vi "SimonGame.vi"() -> ()   [LabVIEW 2024]
uses:
  state machine variables.ctl
  state machine states.ctl
  state machine controller.ctl
panel:
  in  "Button 4":bool
  in  "Button3":bool
  in  "Button 2":bool
  in  "Button 1":bool
  out "Round":dbl
  out "Score":dbl
  # "Score"
  # "Level"
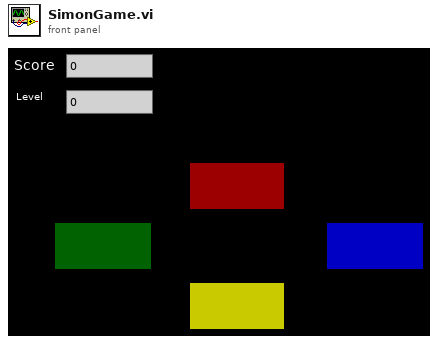
[diagram p1: front panel]
types:
  T1 = typedef "state machine states.ctl" = enum16{"Initialize", "update display", "Show sequence", "User response", "update data", ""}
  T2 = typedef "state machine variables.ctl" = cluster{"Sequence":dbl[], "Score":dbl, "Round":dbl}
  T3 = typedef "VI Communication.ctl" = cluster{"Queue":refnum<queue>, "Path":path, "Score":dbl, "Level":dbl}
  T4 = enum8{"Enabled", "Disabled", "Disabled and Grayed Out"}
  T5 = typedef "state machine controller.ctl" = cluster{"State Machine State":string, "Difficulty":dbl, "Login User Name":string, "Login User Passwd":string}
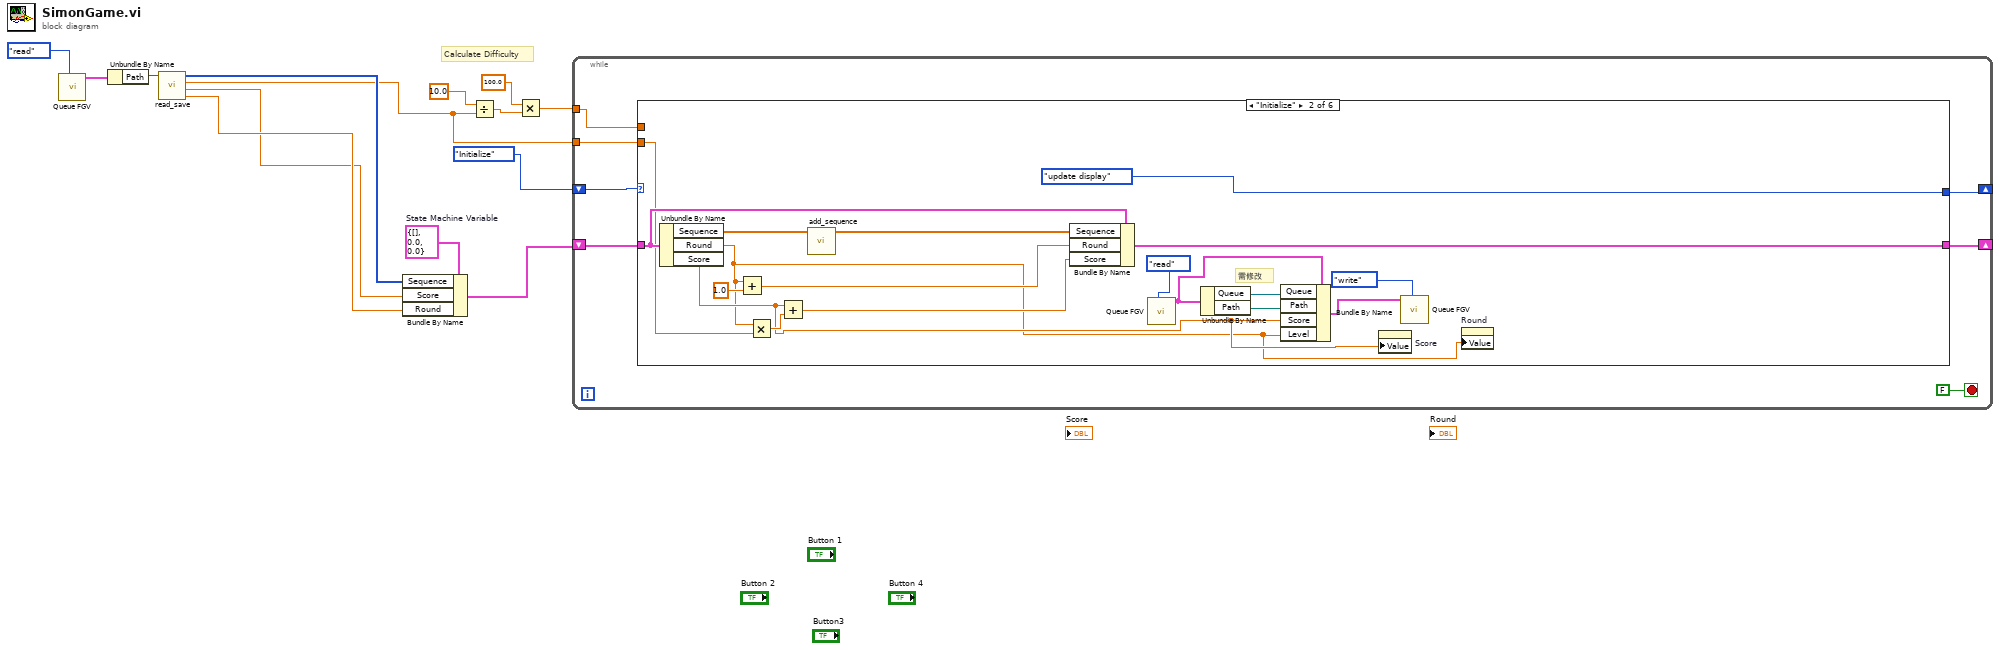
[diagram p0: block diagram]
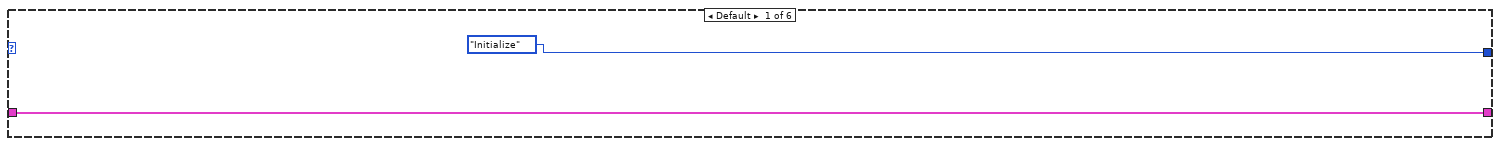
[diagram p2: hidden frame]
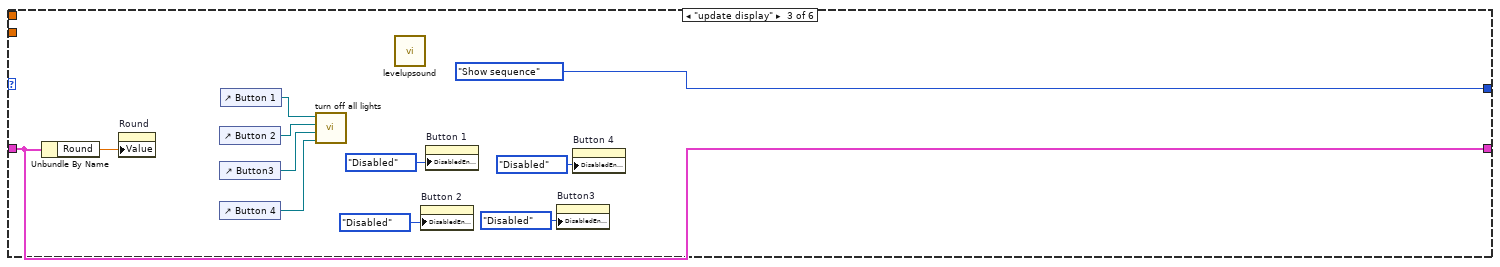
[diagram p3: hidden frame]
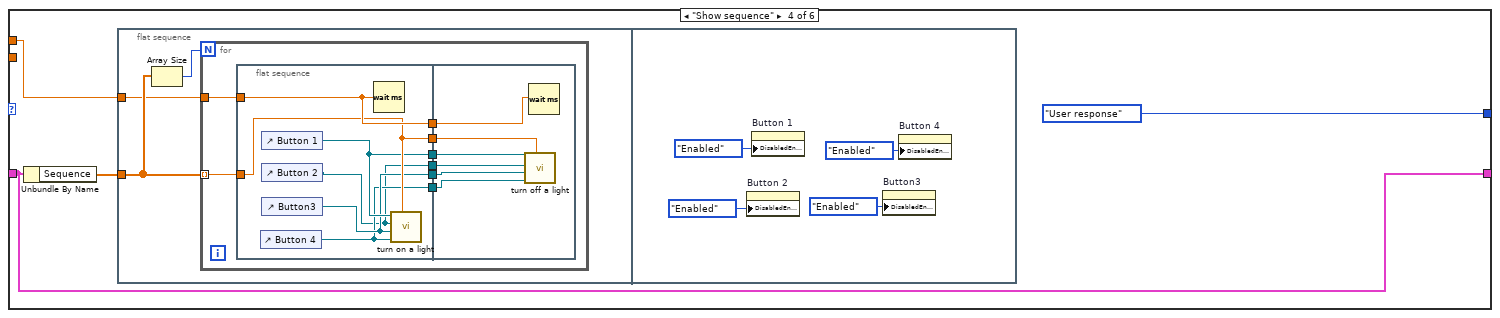
[diagram p4: hidden frame]
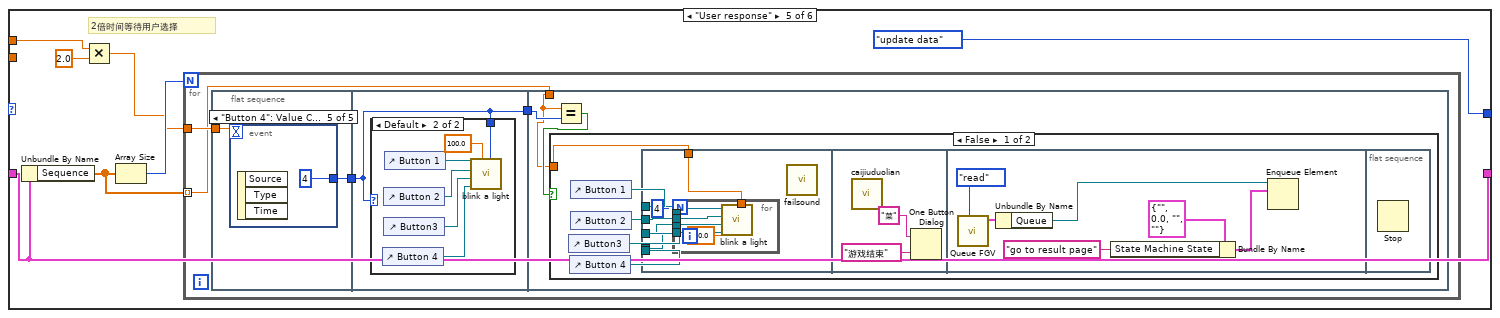
[diagram p5: hidden frame]
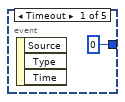
[diagram p6: hidden frame]
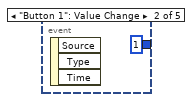
[diagram p7: hidden frame]
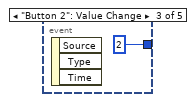
[diagram p8: hidden frame]
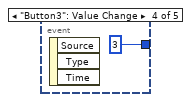
[diagram p9: hidden frame]
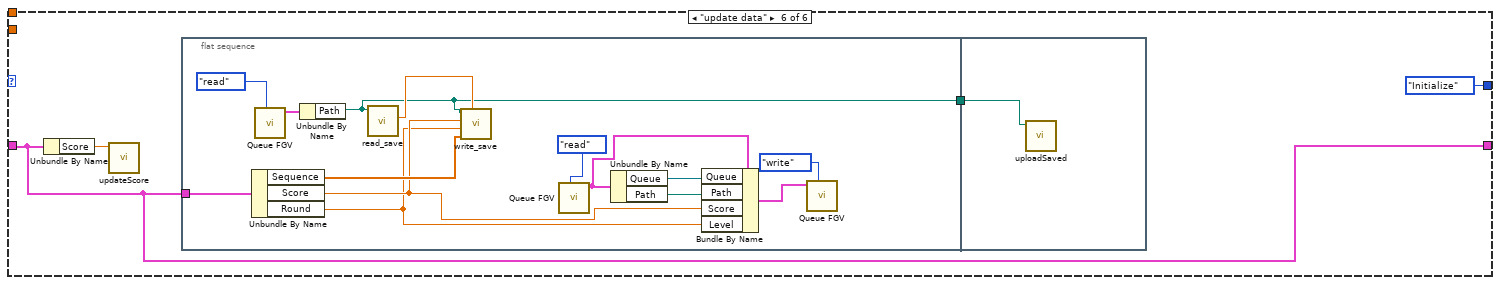
[diagram p12: hidden frame]
diagram:
  w9 = T2 {"Sequence"=[], "Score"=0.0, "Round"=0.0}  # State Machine Variable
  # "Calculate Difficulty"
  n1 = call "Queue FGV.vi"("Enum"=enum16{"read", "write"}."read") -> ("VI Communication Out"=w5:T3)  [unwired: 10 in]
  n2 = Unbundle By Name(w5) -> ("Path"=w4:path)
  n3 = call "read_save.vi"("save file path"=w4) -> ("Level"=w3:dbl, "Score"=w2:dbl, "Difficulty"=w1:dbl, "Sequence Array"=w7:i32[])  [unwired: 6 in, 1 out]
  n4 = Bundle By Name(cluster=w9, "Sequence"=w7, "Score"=w2, "Round"=w3) -> (w8:T2)
  n5 = Divide(x=10.0, y=w1) -> (x/y=w12:dbl)
  n6 = Multiply(x=100.0, y=w12) -> (x*y=w11:dbl)
  n7 = while {
    shift-right: [w17] -> _
    shift-left: w8 -> [w21]
    shift-right: [w19] -> _
    shift-left: state_machine_states."Initialize" -> [w20]
    tunnel: w11 -> [w18]
    tunnel: w1 -> [w16]
    stop <- FALSE stop-if-true
    n8 = case shown="\"Initialize\"" w20 {
      tunnel: w21 -> [w23 w40 w52 w53 w84 w137]
      tunnel: [w23 w39 w52 w53 w84 w137] -> w17
      tunnel: [state_machine_states."Initialize" ("Enum") state_machine_states."update display" ("Enum") state_machine_states."Show sequence" ("Enum") state_machine_states."User response" ("Enum") state_machine_states."update data" ("Enum") state_machine_states."Initialize" ("Enum")] -> w19
      tunnel: w18 -> [_ _ _ w55 w86 _]
      tunnel: w16 -> [_ w34 _ _ _ _]
      frame Default {
      }
      frame "Initialize" {
        # "需修改"
        n9 = Unbundle By Name(w40) -> ("Sequence"=w41:dbl[], "Round"=w24:dbl, "Score"=w25:dbl)
        n10 = Add(x=w24, y=1.0) -> (x+y=w28:dbl)
        n11 = Multiply(x=w24, y=w34) -> (x*y=w35:dbl)
        n12 = Add(x=w25, y=w35) -> (x+y=w27:dbl)
        n13 = call "add_sequence.vi"("sequence in"=w41) -> ("sequence out"=w38:dbl[])  [unwired: 9 in, 1 out]
        n14 = Bundle By Name(cluster=w40, "Sequence"=w38, "Round"=w28, "Score"=w27) -> (w39:T2)
        n15 = call "Queue FGV.vi"("Enum"=enum16{"read", "write"}."read") -> ("VI Communication Out"=w32:T3)  [unwired: 10 in]
        n16 = Unbundle By Name(w32) -> ("Queue"=w30:refnum<queue>, "Path"=w29:path)
        n17 = Bundle By Name(cluster=w32, "Queue"=w30, "Path"=w29, "Score"=w25, "Level"=w24) -> (w26:T3)
        n18 = property on="Score" class="DigNum (strict)"("Value"=w25) -> ()  [unwired: 2 in, 2 out]
        n19 = call "Queue FGV.vi"("Enum"=enum16{"read", "write"}."write", "VI Communication In"=w26) -> ()  [unwired: 9 in, 1 out]
        n20 = property on="Round" class="DigNum (strict)"("Value"=w24) -> ()  [unwired: 2 in, 2 out]
      }
      frame "update display" {
        n21 = Unbundle By Name(w52) -> ("Round"=w51:dbl)
        n22 = property on="Round" class="DigNum (strict)"("Value"=w51) -> ()  [unwired: 2 in, 2 out]
        n23 = control-ref of="Button 2"() -> (w48:refnum<vi>)
        n24 = control-ref of="Button3"() -> (w47:refnum<vi>)
        n25 = control-ref of="Button 4"() -> (w46:refnum<vi>)
        n26 = control-ref of="Button 1"() -> (w49:refnum<vi>)
        n27 = call "turn off all lights.vi"("Button 4"=w46, "Button 3"=w47, "Button 2"=w48, "Button 1"=w49) -> ()  [unwired: 7 in, 1 out]
        n28 = call "levelupsound.vi"() -> ()  [unwired: 11 in, 1 out]
        n29 = property on="Button 2" class="Bool"("DisabledEnum"=T4."Disabled" ("Disabled")) -> ()  [unwired: 2 in, 2 out]
        n30 = property on="Button 1" class="Bool"("DisabledEnum"=T4."Disabled" ("Disabled")) -> ()  [unwired: 2 in, 2 out]
        n31 = property on="Button3" class="Bool"("DisabledEnum"=T4."Disabled" ("Disabled")) -> ()  [unwired: 2 in, 2 out]
        n32 = property on="Button 4" class="Bool"("DisabledEnum"=T4."Disabled" ("Disabled")) -> ()  [unwired: 2 in, 2 out]
      }
      frame "Show sequence" {
        n33 = Unbundle By Name(w53) -> ("Sequence"=w56:dbl[])
        n34 = flat-sequence {
          tunnel: w56 -> [w58]
          tunnel: w55 -> [w57]
          frame #0 {
            n35 = Array Size(array=w58) -> (size(s)=w59:i32)
            n36 = for {
              N: w59 -> [_]
              tunnel: w58 -> [w67] mode=indexing
              tunnel: w57 -> [w66]
              n37 = flat-sequence {
                tunnel: w67 -> [w72]
                tunnel: w66 -> [w73]
                tunnel: [w73] -> w65
                tunnel: [w72] -> w64
                tunnel: [w71] -> w63
                tunnel: [w70] -> w62
                tunnel: [w69] -> w61
                tunnel: [w68] -> w60
                tunnel: w65 -> [w79]
                tunnel: w64 -> [w78]
                tunnel: w63 -> [w77]
                tunnel: w62 -> [w76]
                tunnel: w61 -> [w75]
                tunnel: w60 -> [w74]
                frame #0 {
                  n38 = control-ref of="Button 4"() -> (w69:refnum<vi>)
                  n39 = control-ref of="Button 1"() -> (w71:refnum<vi>)
                  n40 = control-ref of="Button 2"() -> (w68:refnum<vi>)
                  n41 = control-ref of="Button3"() -> (w70:refnum<vi>)
                  n42 = Wait (ms)(milliseconds to wait=w73) -> ()  [unwired: 1 out]
                  n43 = call "turn on a light.vi"("Which Button?"=w72, "Button 4"=w69, "Button 3"=w70, "Button 2"=w68, "Button 1"=w71) -> ()  [unwired: 6 in, 1 out]
                }
                frame #1 {
                  n44 = call "turn off a light.vi"("Which Button?"=w78, "Button 4"=w75, "Button 3"=w76, "Button 2"=w74, "Button 1"=w77) -> ()  [unwired: 6 in, 1 out]
                  n45 = Wait (ms)(milliseconds to wait=w79) -> ()  [unwired: 1 out]
                }
              }
            }
          }
          frame #1 {
            n46 = property on="Button 2" class="Bool"("DisabledEnum"=T4."Enabled" ("Disabled")) -> ()  [unwired: 2 in, 2 out]
            n47 = property on="Button 1" class="Bool"("DisabledEnum"=T4."Enabled" ("Disabled")) -> ()  [unwired: 2 in, 2 out]
            n48 = property on="Button3" class="Bool"("DisabledEnum"=T4."Enabled" ("Disabled")) -> ()  [unwired: 2 in, 2 out]
            n49 = property on="Button 4" class="Bool"("DisabledEnum"=T4."Enabled" ("Disabled")) -> ()  [unwired: 2 in, 2 out]
          }
        }
      }
      frame "User response" {
        # "2倍时间等待用户选择"
        n50 = Unbundle By Name(w84) -> ("Sequence"=w88:dbl[])
        n51 = Multiply(x=w86, y=2.0) -> (x*y=w87:dbl)
        n52 = Array Size(array=w88) -> (size(s)=w89:i32)
        n53 = for {
          N: w89 -> [_]
          tunnel: w88 -> [w92] mode=indexing
          tunnel: w87 -> [w94]
          n54 = flat-sequence {
            tunnel: w94 -> [w96]
            tunnel: [w95] -> w93
            tunnel: w93 -> [w102]
            tunnel: [w102] -> w91
            tunnel: w92 -> [w109]
            tunnel: w91 -> [w111]
            frame #0 {
              n55 = event shown="[4] \"Button 4\": Value Change" {
                selector: _ -> [_ _ _ _ _]
                dyn-events: _ -> [_ _ _ _ _]
                timeout: w96 -> [_ _ _ _ _]
                tunnel: [u32 0 1 2 3 u32 4] -> w95
                event Timeout {
                  n56 = event-data() -> ()  [unwired: 1 in, 3 out]
                }
                event "Button 1": Value Change {
                  n57 = event-data() -> ()  [unwired: 1 in, 3 out]
                }
                event "Button 2": Value Change {
                  n58 = event-data() -> ()  [unwired: 1 in, 3 out]
                }
                event "Button3": Value Change {
                  n59 = event-data() -> ()  [unwired: 1 in, 3 out]
                }
                event "Button 4": Value Change {
                  n60 = event-data() -> ()  [unwired: 1 in, 3 out]
                }
              }
            }
            frame #1 {
              n61 = case shown="Default" w102 {
                tunnel: w102 -> [_ w108]
                frame 0 {
                }
                frame Default {
                  n62 = control-ref of="Button 4"() -> (w104:refnum<vi>)
                  n63 = control-ref of="Button 2"() -> (w106:refnum<vi>)
                  n64 = control-ref of="Button3"() -> (w105:refnum<vi>)
                  n65 = control-ref of="Button 1"() -> (w107:refnum<vi>)
                  n66 = call "blink a light.vi"("Whcih Button?"=w108, "Blink Time"=100.0, "Button 4"=w104, "Button 3"=w105, "Button 2"=w106, "Button 1"=w107) -> ()  [unwired: 5 in, 1 out]
                }
              }
            }
            frame #2 {
              n67 = Equal?(x=w109, y=w111) -> (x = y?=w110:bool)
              n68 = case shown="False" w110 {
                tunnel: w109 -> [w116 _]
                frame False {
                  n69 = control-ref of="Button3"() -> (w113:refnum<vi>)
                  n70 = control-ref of="Button 4"() -> (w112:refnum<vi>)
                  n71 = control-ref of="Button 1"() -> (w115:refnum<vi>)
                  n72 = control-ref of="Button 2"() -> (w114:refnum<vi>)
                  n73 = flat-sequence {
                    tunnel: w116 -> [w122]
                    tunnel: w115 -> [w119]
                    tunnel: w114 -> [w118]
                    tunnel: w113 -> [w120]
                    tunnel: [w121] -> _
                    tunnel: w112 -> [w121]
                    frame #0 {
                      n74 = for {
                        N: 4 -> [_]
                        tunnel: w122 -> [w128]
                        tunnel: w121 -> [w127]
                        tunnel: w120 -> [w126]
                        tunnel: w119 -> [w125]
                        tunnel: w118 -> [w124]
                        n75 = call "blink a light.vi"("Whcih Button?"=w128, "Blink Time"=200.0, "Button 4"=w127, "Button 3"=w126, "Button 2"=w124, "Button 1"=w125) -> ()  [unwired: 5 in, 1 out]
                      }
                      n76 = call "failsound.vi"() -> ()  [unwired: 11 in, 1 out]
                    }
                    frame #1 {
                      n77 = call "caijiuduolian.vi"() -> ()  [unwired: 11 in, 1 out]
                      n78 = One Button Dialog(message="菜", button name ("OK")="游戏结束") -> ()  [unwired: 1 out]
                    }
                    frame #2 {
                      n79 = call "Queue FGV.vi"("Enum"=enum16{"read", "write"}."read") -> ("VI Communication Out"=w131:T3)  [unwired: 10 in]
                      n80 = Unbundle By Name(w131) -> ("Queue"=w135:refnum<queue>)
                      n81 = Bundle By Name(cluster=T5 {"State Machine State"="", "Difficulty"=0.0, "Login User Name"="", "Login User Passwd"=""} ("Cluster"), "State Machine State"="go to result page") -> (w132:T5)
                      n82 = Enqueue Element(queue=w135, element=w132) -> ()  [unwired: 2 in, 3 out]
                    }
                    frame #3 {
                      n83 = Stop() -> ()  [unwired: 1 in]
                    }
                  }
                }
                frame True {
                }
              }
            }
          }
        }
      }
      frame "update data" {
        n84 = Unbundle By Name(w137) -> ("Score"=w140:dbl)
        n85 = call "updateScore.vi"("New Score"=w140) -> ()  [unwired: 10 in, 1 out]
        n86 = flat-sequence {
          tunnel: w137 -> [w152]
          tunnel: [w149] -> w139
          tunnel: w139 -> [w155]
          frame #0 {
            n87 = Unbundle By Name(w152) -> ("Sequence"=w150:dbl[], "Score"=w142:dbl, "Round"=w141:dbl)
            n88 = call "Queue FGV.vi"("Enum"=enum16{"read", "write"}."read") -> ("VI Communication Out"=w153:T3)  [unwired: 10 in]
            n89 = Unbundle By Name(w153) -> ("Path"=w149:path)
            n90 = call "read_save.vi"("save file path"=w149) -> ("Difficulty"=w151:dbl)  [unwired: 6 in, 4 out]
            n91 = call "write_save.vi"("Difficulty"=w151, "Sequence"=w150, "Level"=w141, "Score"=w142, "save file path"=w149) -> ()  [unwired: 6 in, 1 out]
            n92 = call "Queue FGV.vi"("Enum"=enum16{"read", "write"}."read") -> ("VI Communication Out"=w147:T3)  [unwired: 10 in]
            n93 = Unbundle By Name(w147) -> ("Queue"=w144:refnum<queue>, "Path"=w143:path)
            n94 = Bundle By Name(cluster=w147, "Queue"=w144, "Path"=w143, "Score"=w142, "Level"=w141) -> (w146:T3)
            n95 = call "Queue FGV.vi"("Enum"=enum16{"read", "write"}."write", "VI Communication In"=w146) -> ()  [unwired: 9 in, 1 out]
          }
          frame #1 {
            n96 = call "uploadSaved.vi"("Path"=w155) -> ()  [unwired: 10 in, 1 out]
          }
        }
      }
    }
  }
